vi "Main.vi"() -> ()   [LabVIEW 2017]
doc: "Use this template to build a user interface event handler design pattern. Use this pattern for dialog boxes and other user interfaces. You also can create and execute user-defined events that the VI can handle the same way as user interface events."
uses:
  <vilib>/Utility/NIReport.llb/HTML Report Image Alignment.ctl
  <vilib>/Utility/NIReport.llb/image depth.ctl
  <vilib>/addons/database/Connection.llb/DB Tools Open Connec (Path).vi
  <vilib>/addons/database/Auxilliary.llb/DB Tools Format Datetime String (Time Stamp).vi
  GLOBAL/auto.vi
  <vilib>/Utility/NIReport.llb/Append Report Text (str wrap).vi
  <vilib>/Utility/NIReport.llb/NI_report.lvclass
  <vilib>/addons/database/NI_Database_API.lvlib
  <vilib>/Utility/NIReport.llb/NI_ReportGenerationCore.lvlib
  <vilib>/Utility/NIReport.llb/Excel/NI_Excel.lvclass
panel:
  out "columns":string[](array[string])
  in  "MAX MIN VALUES":enum32{"ACTUAL", "SET"}(tab)
  out "TEMP":cluster{"MIN":dbl, "MAX":dbl, "ACTUAL":dbl}
  out "FLOW":cluster{"MIN":dbl, "MAX":dbl, "ACTUAL":dbl}
  out "BMP":cluster{"ACTUAL":dbl}
  out "Pressure":cluster{"MIN":dbl, "MAX":dbl, "ACTUAL":dbl}
  out "TEMP SET":cluster{"MIN":dbl, "MAX":dbl, "THRESHOLD":dbl}
  out "FLOW SET":cluster{"MIN":dbl, "MAX":dbl, "THRESHOLD":dbl}
  out "BMP SET":cluster{"MIN":dbl, "MAX":dbl, "THRESHOLD":dbl}
  out "Pressure SET":cluster{"MIN":dbl, "MAX":dbl, "THRESHOLD":dbl}
  out "Loading....":u8(slide) scale=0.0..100.0
  out "BMP":bool
  out "Temp":bool
  out "Flow":bool
  out "Pressure":bool
  in  "Generate Report":bool
  out "DESCRIPTION":string
  out "resulting string":path
  in  "import state 3":bool
  out "User Name":string
  out "Min Peak/Min":dbl
  out "Status bar":string
  in  "import state 2":bool
  out "SELECTED RECIPE":string
  out "BARCODE_FOUND":bool
  out "DB CONN":bool
  in  "Graph":bool
  out "table":string[][](table)
  out "GRAPH":cluster{timestamp[], ext[]}[](graph)
  out "TEST RESULT":bool
  in  "BARCODE":string
  out "SELECTED FILE PATH":path
  in  "Import File":bool
  in  "SELECT MEASURED FILE":i32(listbox)
  out "error out":errorcluster
  in  "File Name":string
  in  "Report Files Folder":path
  in  "Convert":bool
  in  "BROWSE FILE FOLDER":path
  in  "stop":bool
  # "Main"
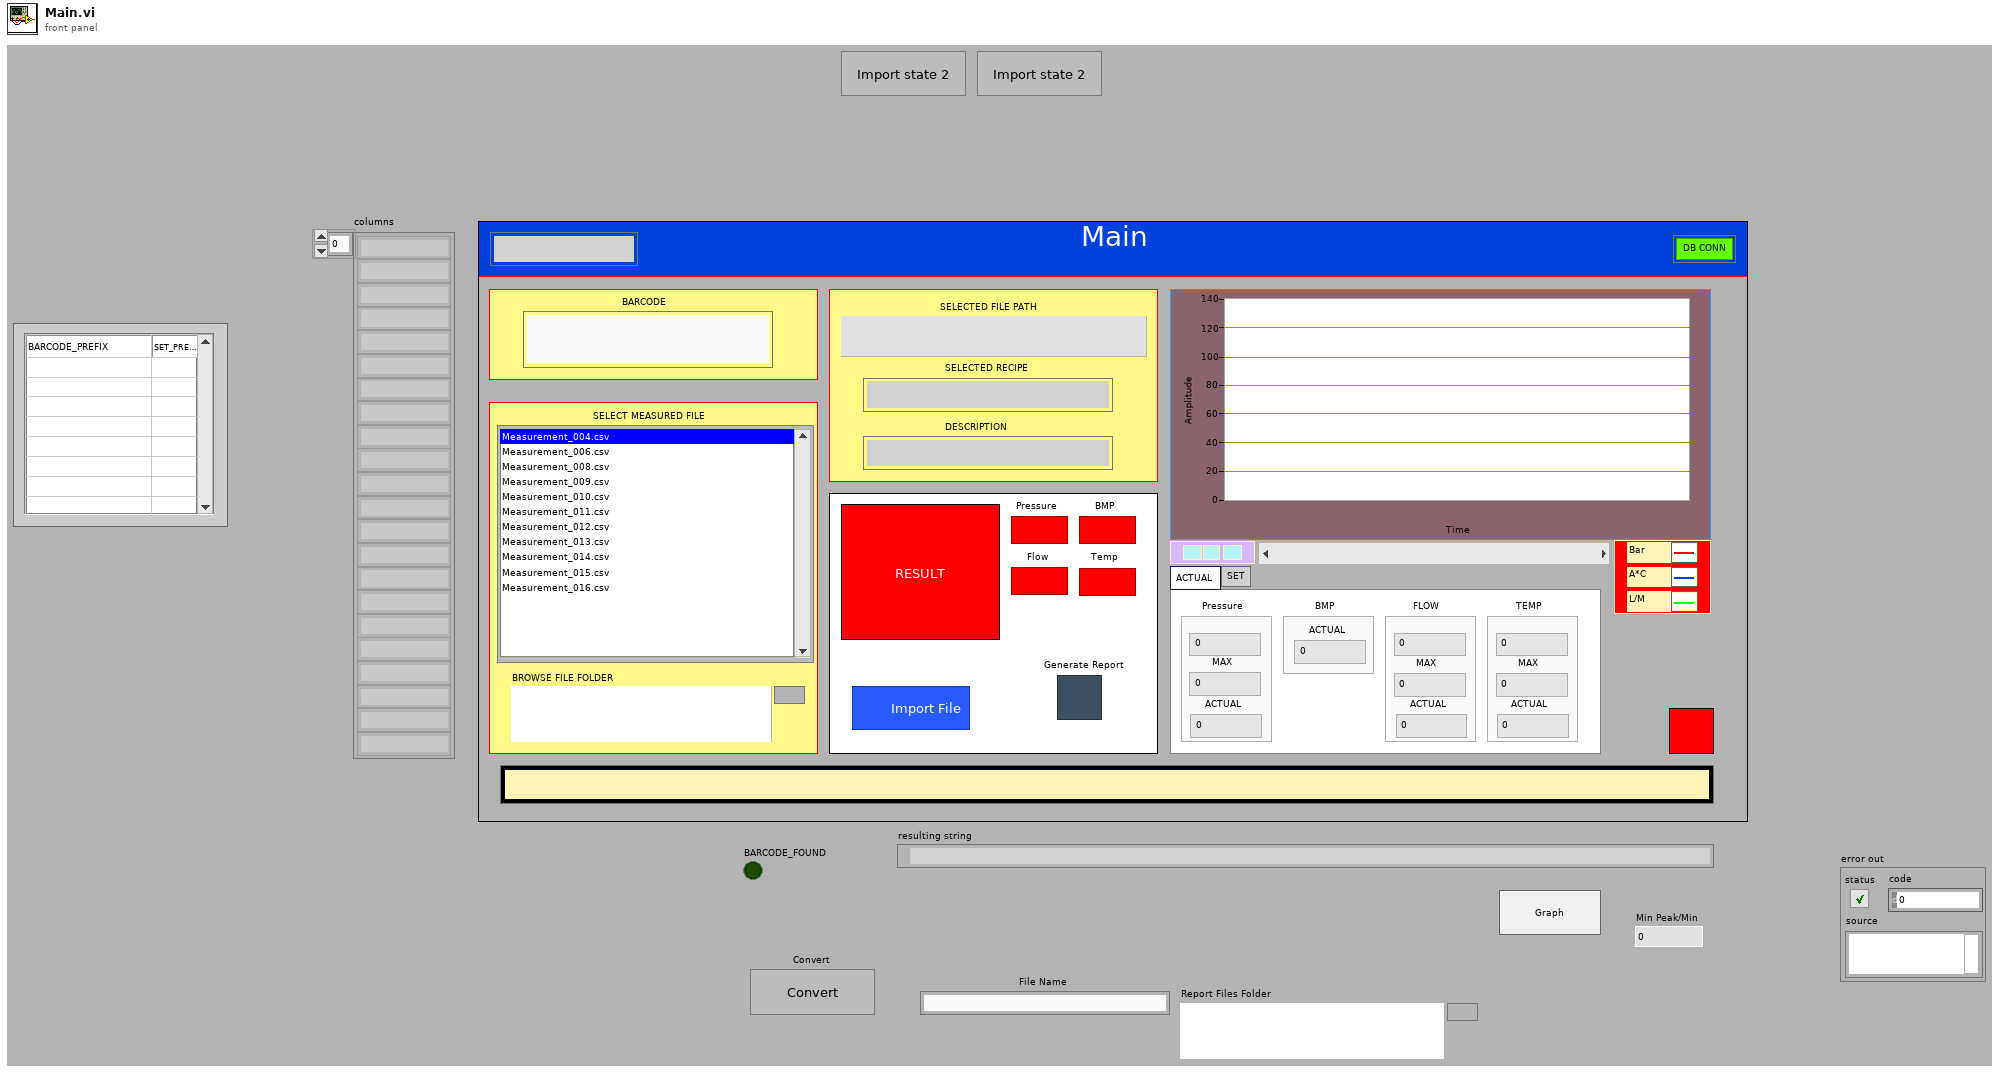
[diagram p1: front panel]
types:
  T1 = cluster{"Files":string[], "Browse File":path, "TIMEOUT":i32, "GRAPH":cluster{timestamp[], ext[]}[], "Pressure":cluster{"chl1 MIN":dbl, "chl1 MAX":dbl, "chl1 thrshold":dbl}, "Flow":cluster{"chl2 MIN":dbl, "chl2 MAX":dbl, "chl2 thrshold":dbl}, "Temp":cluster{"chl3 MIN":dbl, "chl3 MAX":dbl, "chl3 thrshold":dbl}, "Report File":path, "Data_to_report":cluster{"date/time string":string, "User Name":string, "BARCODE":string, "SELECTED RECIPE":string, "Rst":string, "Error Code":string, "RESULT ARRAY":string[]}, "BMP":cluster{"chl3 MIN":dbl, "chl3 MAX":dbl, "chl3 thrshold":dbl}}
  T2 = typedef "NI_Database_API.lvlib/Conn ObjectReference.ctl" = refnum<k1>
  T3 = enum32{"Invalid", "Standard", "Closed", "Hidden", "Minimized", "Maximized"}
  T4 = cluster{"position (Excel)":cluster{"row":i32, "column":i32}, "name (Excel)":string, "bookmark (Word)":string}[]
  T5 = cluster{"position (Excel)":cluster{"row":i32, "column":i32}, "name (Excel)":string, "bookmark (Word)":string}
  T6 = typedef "NI_ReportGenerationCore.lvlib/HTML Report Image Alignment.ctl" = enum16{"(default)", "LEFT", "RIGHT", "TOP", "TEXTTOP", "MIDDLE", "ABSMIDDLE", "BASELINE", "BOTTOM", "ABSBOTTOM"}
  T7 = enum16{"Standard Report", "HTML", "Word", "Excel"}
  T8 = enum16{"maximized", "minimized", "normal", "no change"}
  T9 = cluster{"Pressure":cluster{"chl1 MIN":dbl, "chl1 MAX":dbl, "chl1 thrshold":dbl}, "Flow":cluster{"chl2 MIN":dbl, "chl2 MAX":dbl, "chl2 thrshold":dbl}, "Temp":cluster{"chl3 MIN":dbl, "chl3 MAX":dbl, "chl3 thrshold":dbl}, "BMP":cluster{"chl3 MIN":dbl, "chl3 MAX":dbl, "chl3 thrshold":dbl}}
  T10 = cluster{"chl1 MIN":dbl, "chl1 MAX":dbl, "chl1 thrshold":dbl}
  T11 = cluster{"chl2 MIN":dbl, "chl2 MAX":dbl, "chl2 thrshold":dbl}
  T12 = cluster{"chl3 MIN":dbl, "chl3 MAX":dbl, "chl3 thrshold":dbl}
  T13 = cluster{"date/time string":string, "User Name":string, "BARCODE":string, "SELECTED RECIPE":string, "Rst":string, "Error Code 2":string}
  T14 = cluster{"date/time string":string, "User Name":string, "BARCODE":string, "SELECTED RECIPE":string, "Rst":string, "Error Code 2":string, "element":string, "element":string, "element":string, "element":string, "element":string, "element":string, "element":string, "element":string, "element":string, "element":string, "element":string}
  T15 = cluster{"date/time string":string, "User Name":string, "BARCODE":string, "SELECTED RECIPE":string, "Rst":string, "Error Code 2":string, "RESULT ARRAY":string[]}
  T16 = typedef "NI_ReportGenerationCore.lvlib/image depth.ctl" = u16
  T17 = enum32{"invalid app kind", "Development System", "Run Time System", "Student Edition", "Embedded LabVIEW", "Evaluation", "Custom"}
  T18 = cluster{"date/time string":string, "User Name":string, "BARCODE":string, "SELECTED RECIPE":string, "Rst":string, "Error Code":string, "RESULT ARRAY":string[]}
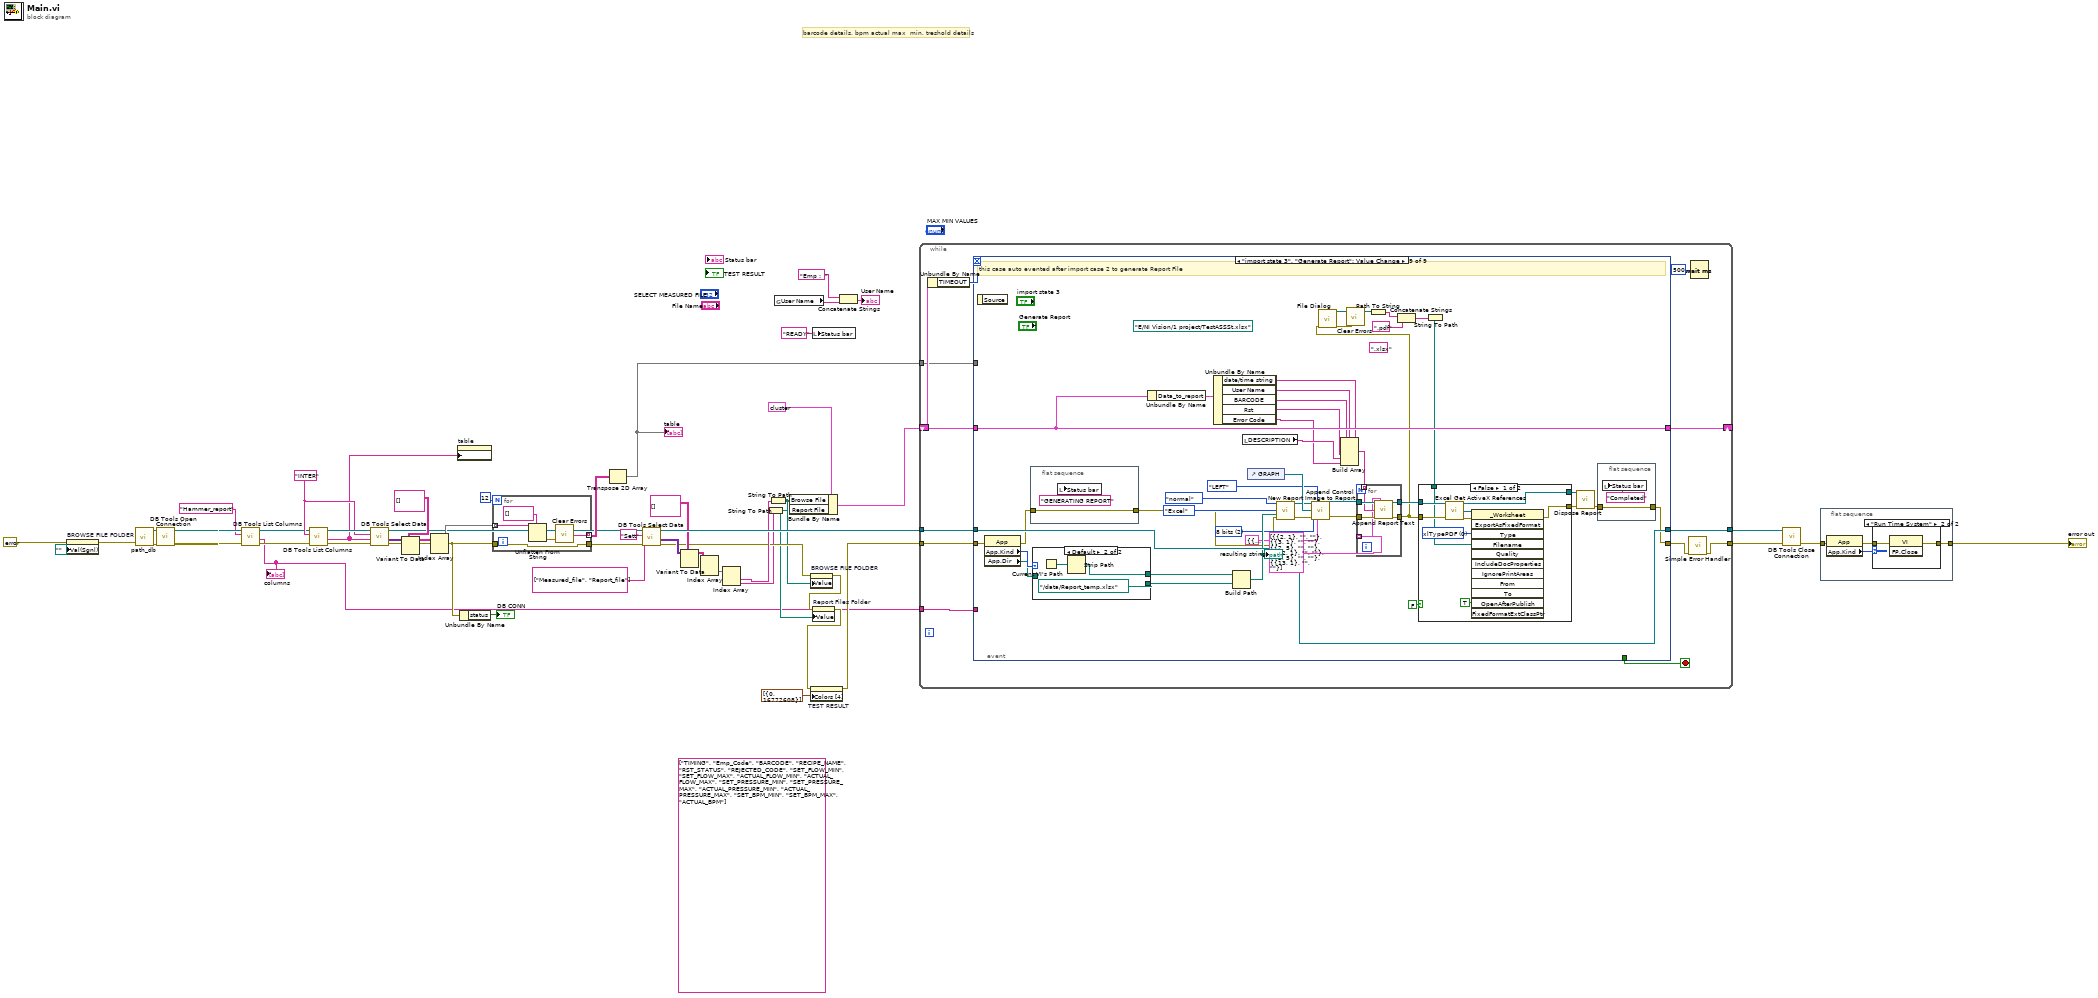
[diagram p0: block diagram]
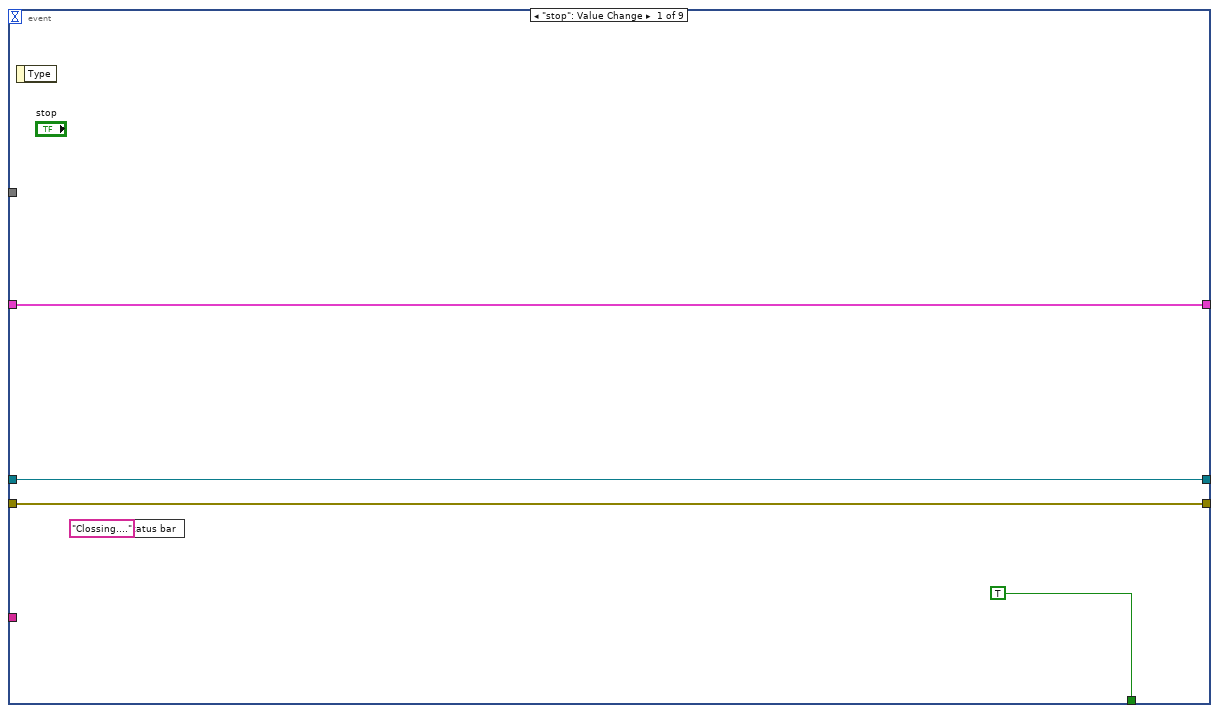
[diagram p3: hidden frame]
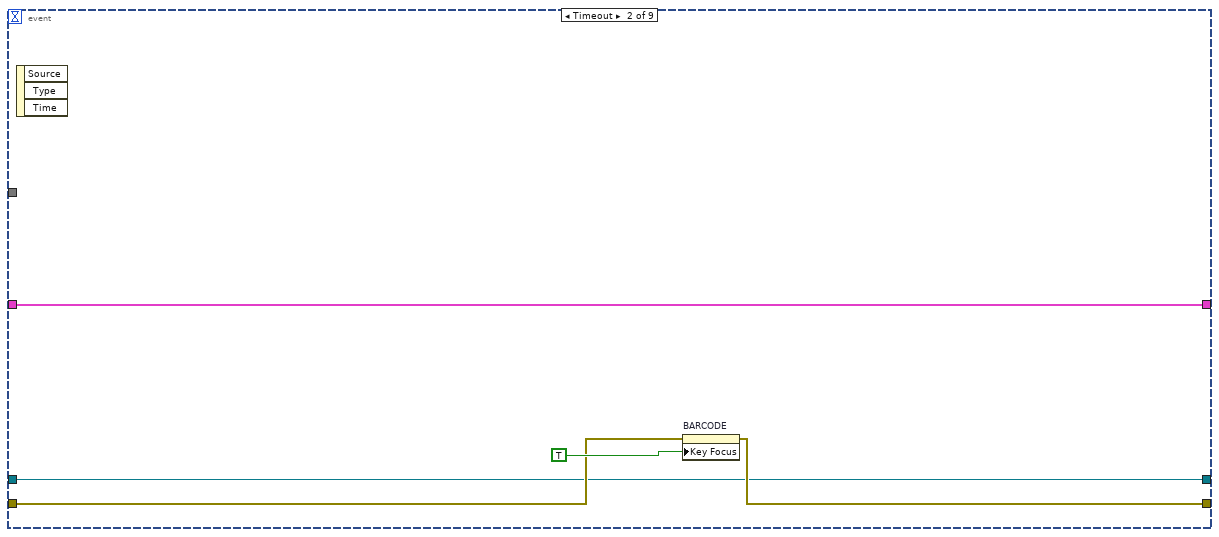
[diagram p4: hidden frame]
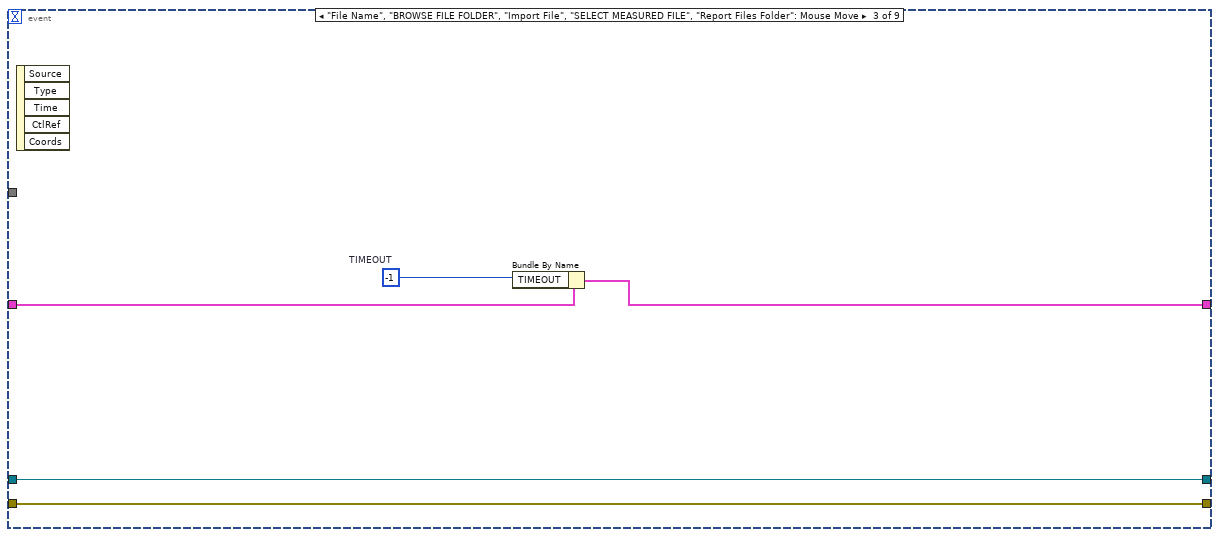
[diagram p5: hidden frame]
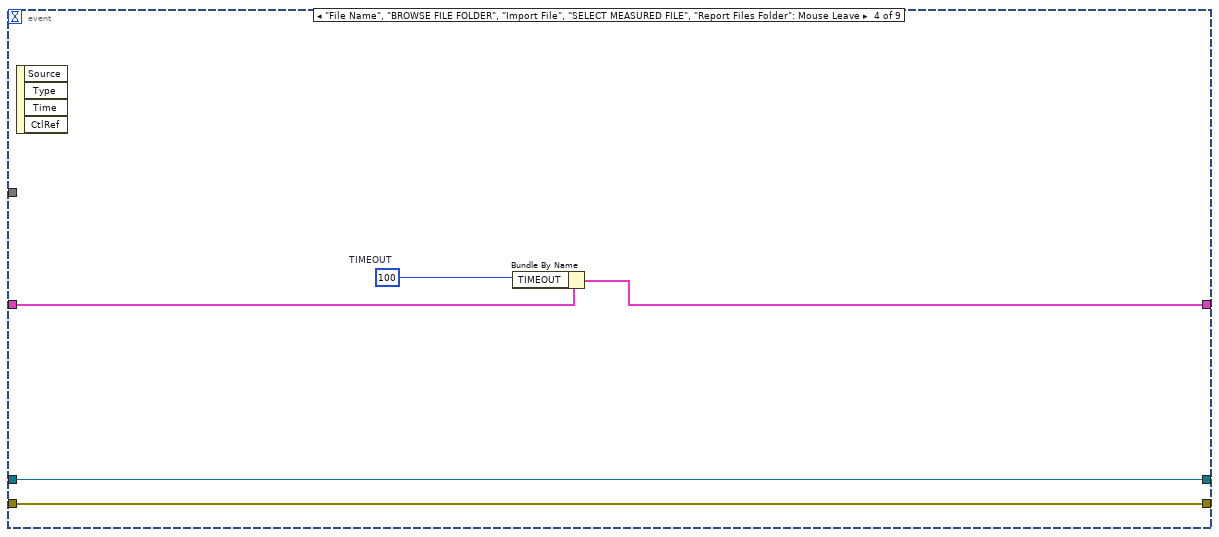
[diagram p6: hidden frame]
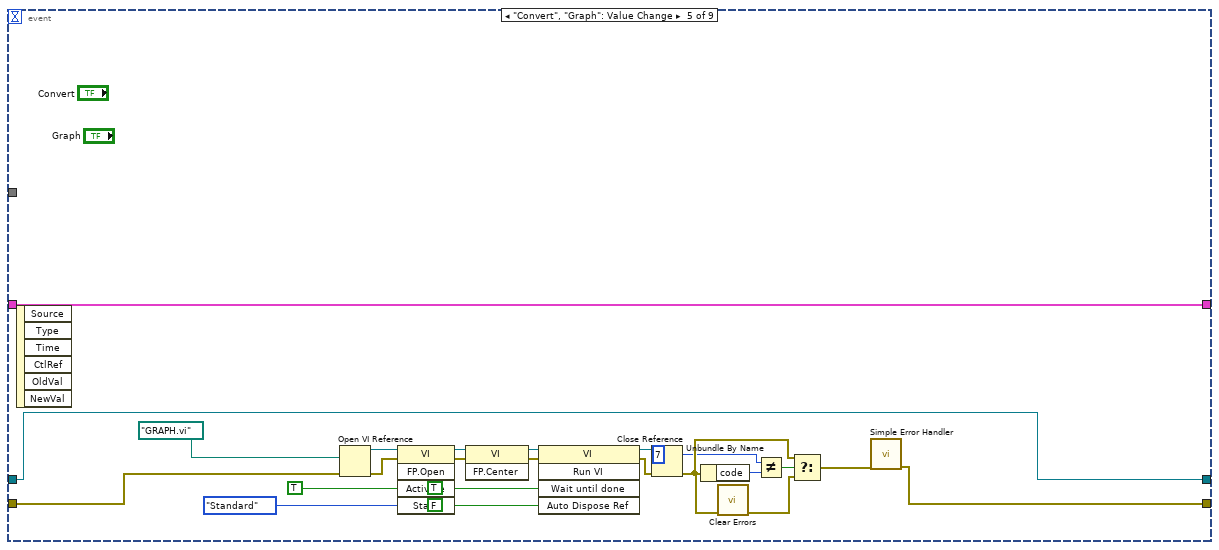
[diagram p7: hidden frame]
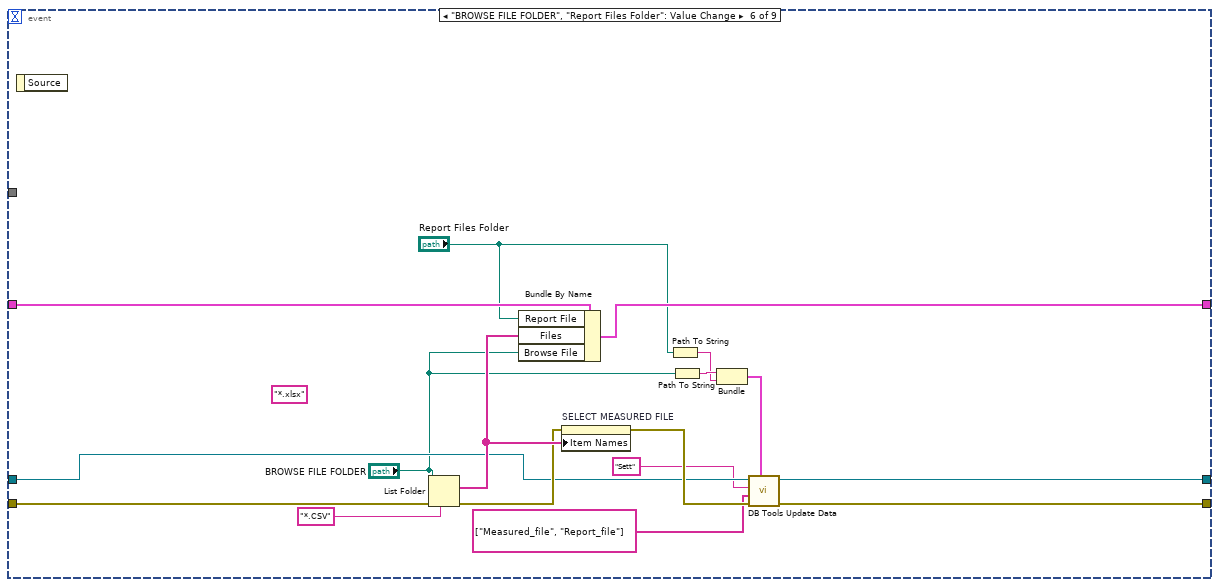
[diagram p8: hidden frame]
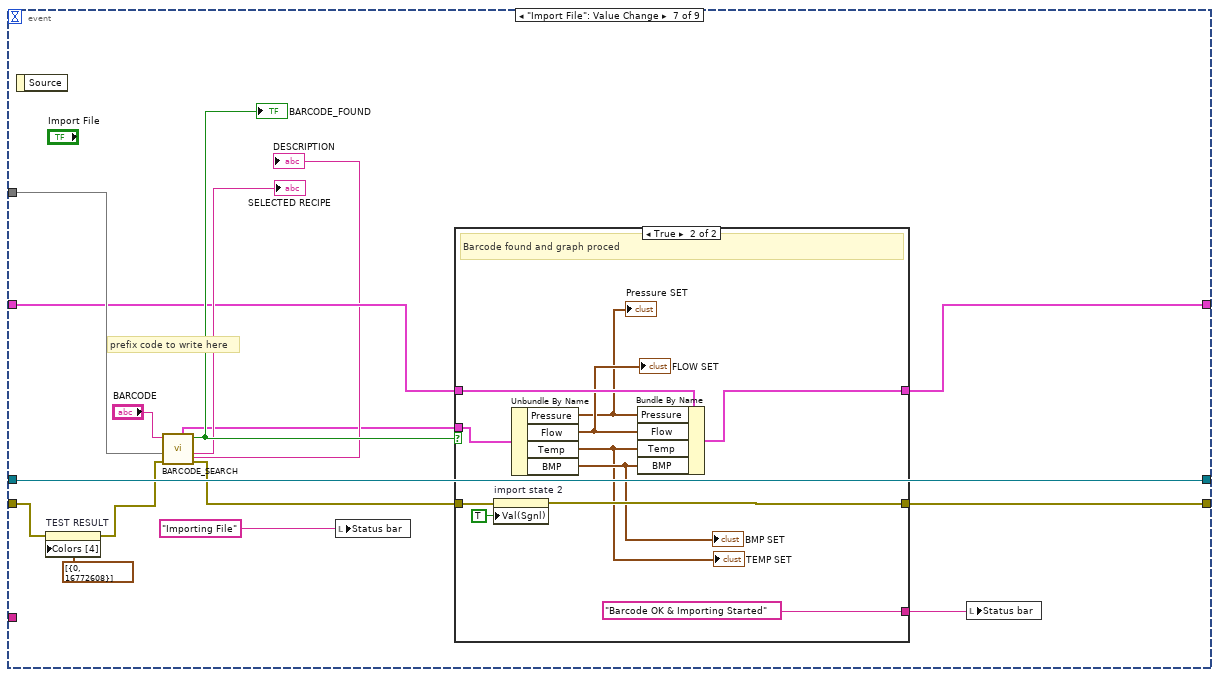
[diagram p9: hidden frame]
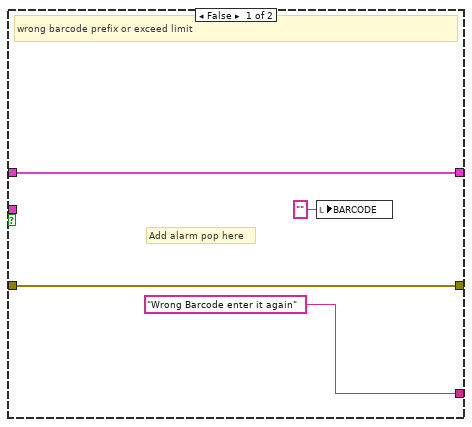
[diagram p10: hidden frame]
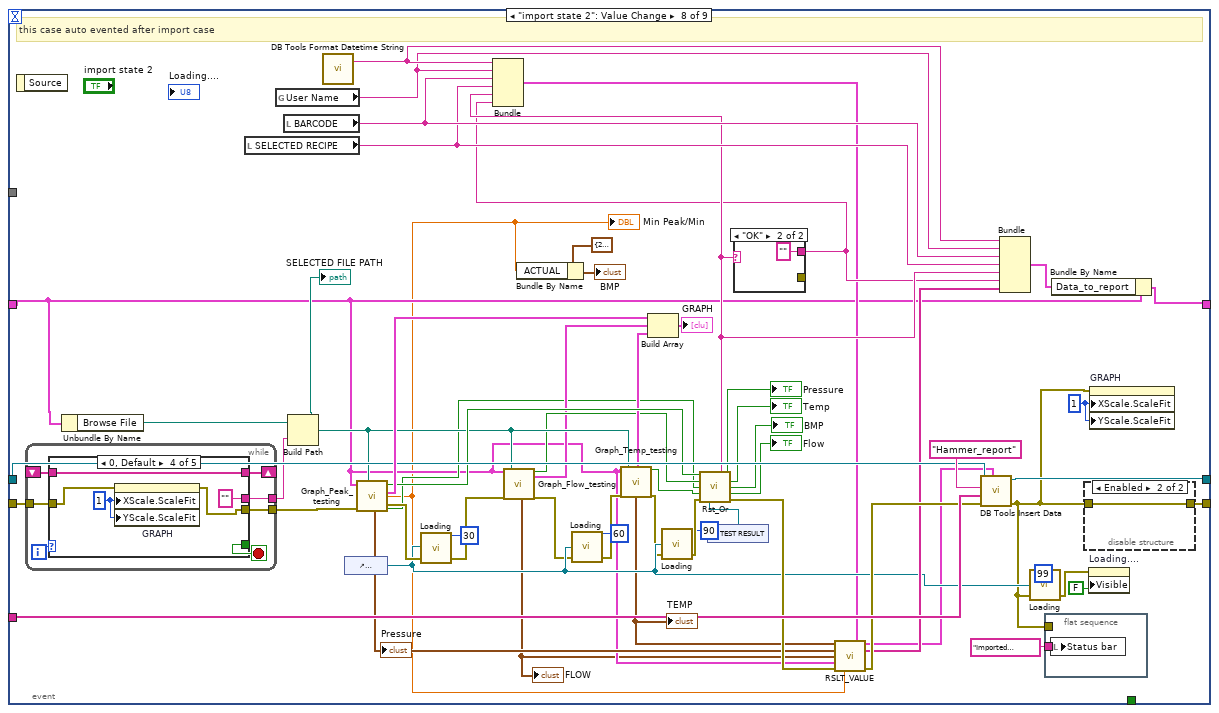
[diagram p11: hidden frame]
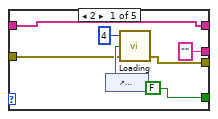
[diagram p12: hidden frame]
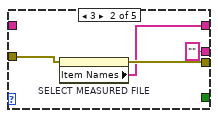
[diagram p13: hidden frame]
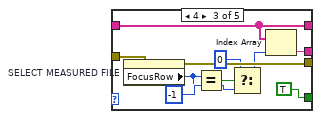
[diagram p14: hidden frame]
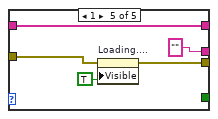
[diagram p15: hidden frame]
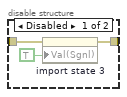
[diagram p16: hidden frame]
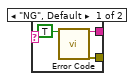
[diagram p17: hidden frame]
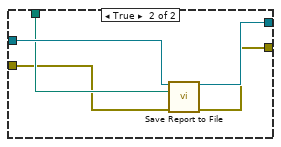
[diagram p18: hidden frame]
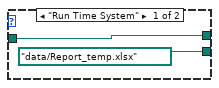
[diagram p19: hidden frame]
diagram:
  (unwired) string[] ["TIMING", "Emp_Code", "BARCODE", "RECIPE_NAME", "RST_STATUS", "REJECTED_CODE", "SET_FLOW_MIN", "SET_FLOW_MAX", "ACTUAL_FLOW_MIN", "ACTUAL_FLOW_MAX", "SET_PRESSURE_MIN", "SET_PRESSURE_MAX", "ACTUAL_PRESSURE_MIN", "ACTUAL_PRESSURE_MAX", "SET_BPM_MIN", "SET_BPM_MAX", "ACTUAL_BPM"] ("columns")
  w11 = "INTER" ("table")
  # "barcode details, bpm actual max  min, treshold details"
  n1 = property on="BROWSE FILE FOLDER" class="Path"(error in=errorcluster {"status"=FALSE, "code"=0, "source"=""} ("error out 2"), "Val(Sgnl)"=path "" ("BROWSE FILE FOLDER")) -> (error out=w25:errorcluster)  [unwired: 1 in, 1 out]
  n2 = call "path_db.vi"("error in"=w25) -> ("error out"=w49:errorcluster, "resulting string"=w48:path)  [unwired: 9 in]
  n3 = call-poly <vilib>:"DB Tools Open Connection.vi"("error in (no error)"=w49, "connection information"=w48) -> ("error out"=w9:errorcluster, "connection reference"=w7:T2)  [unwired: 6 in]
  n4 = call <vilib>:"DB Tools List Columns.vi"("error in (no error)"=w9, "table"="Hammer_report", "connection reference"=w7) -> ("error out"=w8:errorcluster, "columns"=w4:string[], "connection reference out"=w6:T2)  [unwired: 1 in, 1 out]
  "columns" <- w4
  n5 = call <vilib>:"DB Tools List Columns.vi"("error in (no error)"=w8, "table"=w11, "connection reference"=w6) -> ("error out"=w13:errorcluster, "columns"=w1:string[], "connection reference out"=w12:T2)  [unwired: 1 in, 1 out]
  n6 = call <vilib>:"DB Tools Select Data.vi"("error in (no error)"=w13, "columns"=w1, "table"=w11, "connection reference"=w12) -> ("error out"=w43:errorcluster, "data"=w51:variant[][], "connection reference out"=w38:T2)  [unwired: 2 in]
  n7 = Variant To Data(type=string[][] [], Variant=w51) -> (data=w50:string[][])  [unwired: 1 in, 1 out]
  n8 = Index Array(array=w50) -> (element=w46:string[])  [unwired: 2 in]
  n9 = property on="table" class="Tbl (strict)"("Column Headers[]"=w1) -> ()  [unwired: 2 in, 2 out]
  n10 = Unbundle By Name(w43) -> ("status"=→"DB CONN":bool)
  n11 = for {
    N: 12 -> [_]
    tunnel: w46 -> [w56] mode=indexing
    tunnel: [w54] -> w45 mode=indexing
    tunnel: w43 -> [w53]
    tunnel: [w53] -> w39
    n12 = Unflatten From String(type=string[] [], binary string=w56) -> (value=w54:string[], error out=w57:errorcluster)  [unwired: 3 in, 1 out]
    n13 = call <vilib>:"Clear Errors.vi"("error in (no error)"=w57) -> ()  [unwired: 5 in, 2 out]
  }
  n14 = Transpose 2D Array(2D array=w45) -> (transposed array=w23:string[][])
  "table" <- w23
  n15 = call <vilib>:"DB Tools Select Data.vi"("error in (no error)"=w39, "columns"=string[] ["Measured_file", "Report_file"], "table"="Sett", "connection reference"=w38) -> ("error out"=w28:errorcluster, "data"=w36:variant[][], "connection reference out"=w37:T2)  [unwired: 2 in]
  n16 = Variant To Data(type=string[][] [], Variant=w36) -> (data=w34:string[][])  [unwired: 1 in, 1 out]
  n17 = Index Array(array=w34) -> (element=w30:string[])  [unwired: 2 in]
  n18 = Index Array(array=w30) -> (element #1=w29:string, element #2=w22:string)  [unwired: 2 in]
  n19 = String To Path(string=w22) -> (path=w21:path)
  n20 = String To Path(string=w29) -> (path=w27:path)
  n21 = global read "auto.vi" "User Name"() -> (w3:string)
  n22 = Bundle By Name(cluster=T1 {"Files"=[], "Browse File"=path "", "TIMEOUT"=100, "GRAPH"=[{array[68443 elements], array[68443 elements]}, {array[68363 elements], array[68363 elements]}, {array[40500 elements], array[40500 elements]}], "Pressure"={"chl1 MIN"=110.0, "chl1 MAX"=130.0, "chl1 thrshold"=120.0}, "Flow"={"chl2 MIN"=33.0, "chl2 MAX"=35.0, "chl2 thrshold"=25.0}, "Temp"={"chl3 MIN"=20.0, "chl3 MAX"=30.0, "chl3 thrshold"=34.0}, "Report File"=path "", "Data_to_report"={"date/time string"="", "User Name"="", "BARCODE"="", "SELECTED RECIPE"="", "Rst"="", "Error Code"="", "RESULT ARRAY"=[]}, "BMP"={"chl3 MIN"=1000.0, "chl3 MAX"=2000.0, "chl3 thrshold"=0.0}}, "Browse File"=w27, "Report File"=w21) -> (w31:T1)
  n23 = property on="BROWSE FILE FOLDER" class="Path"(error in=w28, "Value"=w27) -> (error out=w20:errorcluster)  [unwired: 1 in, 1 out]
  n24 = local write "Status bar"("READY" ("Status bar")) -> ()
  n25 = property on="Report Files Folder" class="Path"(error in=w20, "Value"=w21) -> (error out=w19:errorcluster)  [unwired: 1 in, 1 out]
  n26 = property on="TEST RESULT" class="Bool"(error in=w19, "Colors [4]"=cluster{u32, u32}[] [{0, 16772608}]) -> (error out=w15:errorcluster)  [unwired: 1 in, 1 out]
  n27 = Concatenate Strings("Emp :  " ("string"), w3) -> (→"User Name":string)
  n28 = while {
    tunnel: w15 -> [w67]
    tunnel: [w59] -> w42
    shift-right: [w66] -> _
    shift-left: w31 -> [w64]
    tunnel: w37 -> [w62]
    tunnel: [w63] -> w41
    tunnel: w23 -> [w61]
    tunnel: w4 -> [w58]
    stop <- w69 stop-if-true
    n29 = Unbundle By Name(w64) -> ("TIMEOUT"=w65:i32)
    n30 = event shown="[8] \"import state 3\", \"Generate Report\": Value Change" {
      selector: _ -> [_ _ _ _ _ _ _ _ _]
      dyn-events: _ -> [_ _ _ _ _ _ _ _ _]
      timeout: w65 -> [_ _ _ _ _ _ _ _ _]
      tunnel: [TRUE _ _ _ _ _ _ _ _] -> w69
      tunnel: w67 -> [w73 w77 w84 w89 w92 w129 w135 w196 w303]
      tunnel: [w73 w76 w84 w89 w91 w122 w142 w213 w285] -> w60
      tunnel: w64 -> [w74 w79 w83 w88 w112 w128 w138 w167 w291]
      tunnel: [w74 w79 w82 w87 w112 w127 w137 w212 w291] -> w66
      tunnel: [w71 w75 w80 w85 w90 w120 w145 w214 w308] -> w63
      tunnel: w62 -> [w71 w75 w80 w85 w90 w121 w145 w215 w308]
      tunnel: w61 -> [_ _ _ _ _ _ w139 _ _]
      tunnel: w58 -> [_ _ _ _ _ _ _ w210 _]
      event "stop": Value Change {
        n31 = event-data() -> ()  [unwired: 1 in, 1 out]
        n32 = local write "Status bar"("Clossing...." ("Status bar")) -> ()
      }
      event Timeout {
        n33 = event-data() -> ()  [unwired: 1 in, 3 out]
        n34 = property on="BARCODE" class="Str"(error in=w77, "Key Focus"=TRUE) -> (error out=w76:errorcluster)  [unwired: 1 in, 1 out]
      }
      event "File Name", "BROWSE FILE FOLDER", "Import File", "SELECT MEASURED FILE", "Report Files Folder": Mouse Move {
        w81 = -1  # TIMEOUT
        n35 = event-data() -> ()  [unwired: 1 in, 5 out]
        n36 = Bundle By Name(cluster=w83, "TIMEOUT"=w81) -> (w82:T1)
      }
      event "File Name", "BROWSE FILE FOLDER", "Import File", "SELECT MEASURED FILE", "Report Files Folder": Mouse Leave {
        w86 = 100  # TIMEOUT
        n37 = event-data() -> ()  [unwired: 1 in, 4 out]
        n38 = Bundle By Name(cluster=w88, "TIMEOUT"=w86) -> (w87:T1)
      }
      event "Convert", "Graph": Value Change {
        n39 = event-data() -> ()  [unwired: 1 in, 6 out]
        n40 = Open VI Reference(vi path=path "GRAPH.vi", error in (no error)=w92) -> (vi reference=w99:refnum<vi>, error out=w111:errorcluster)  [unwired: 4 in]
        n41 = invoke class="VI" method="FP.Open"(reference=w99, error in=w111, "Activate"=TRUE ("Activate?"), "State"=T3."Standard") -> (reference out=w110:refnum<vi>, error out=w105:errorcluster)  [unwired: 1 in, 3 out]
        n42 = invoke class="VI" method="FP.Center"(reference=w110, error in=w105) -> (reference out=w106:refnum<vi>, error out=w107:errorcluster)  [unwired: 1 in, 1 out]
        n43 = invoke class="VI" method="Run VI"(reference=w106, error in=w107, "Wait until done"=TRUE ("Wait Until Done"), "Auto Dispose Ref"=FALSE ("Auto Dispose Reference")) -> (reference out=w108:refnum<vi>, error out=w109:errorcluster)  [unwired: 1 in, 3 out]
        n44 = Close Reference(reference=w108, error in (no error)=w109) -> (error out=w100:errorcluster)
        n45 = Unbundle By Name(w100) -> ("code"=w104:i32)
        n46 = call <vilib>:"Clear Errors.vi"("error in (no error)"=w100) -> ("error out"=w102:errorcluster)  [unwired: 5 in, 1 out]
        n47 = Not Equal?(x=7, y=w104) -> (x != y?=w103:bool)
        n48 = Select(t=w100, s=w103, f=w102) -> (s? t:f=w101:errorcluster)
        n49 = call <vilib>:"Simple Error Handler.vi"("error in (no error)"=w101) -> ("error out"=w91:errorcluster)  [unwired: 4 in, 4 out]
      }
      event "BROWSE FILE FOLDER", "Report Files Folder": Value Change {
        (unwired) "*.xlsx" ("pattern")
        n50 = event-data() -> ()  [unwired: 1 in, 1 out]
        n51 = List Folder(path="BROWSE FILE FOLDER", pattern="*.CSV", error in=w129) -> (filenames=w125:string[], error out=w124:errorcluster)  [unwired: 1 in, 2 out]
        n52 = Bundle By Name(cluster=w128, "Report File"="Report Files Folder", "Files"=w125, "Browse File"="BROWSE FILE FOLDER") -> (w127:T1)
        n53 = property on="SELECT MEASURED FILE" class="LstBox (strict)"(error in=w124, "Item Names"=w125) -> (error out=w123:errorcluster)  [unwired: 1 in, 1 out]
        n54 = Path To String(path="Report Files Folder") -> (string=w114:string)
        n55 = Path To String(path="BROWSE FILE FOLDER") -> (string=w116:string)
        n56 = Bundle(w116, w114) -> (w119:cluster{string, string})  [unwired: 1 in]
        n57 = call <vilib>:"DB Tools Update Data.vi"("data"=w119, "error in (no error)"=w123, "columns"=string[] ["Measured_file", "Report_file"], "table"="Sett", "connection reference"=w121) -> ("error out"=w122:errorcluster, "connection reference out"=w120:T2)  [unwired: 5 in]
      }
      event "Import File": Value Change {
        # "prefix code to write here"
        n58 = event-data() -> ()  [unwired: 1 in, 1 out]
        n59 = property on="TEST RESULT" class="Bool"(error in=w135, "Colors [4]"=cluster{u32, u32}[] [{0, 16772608}]) -> (error out=w134:errorcluster)  [unwired: 1 in, 1 out]
        n60 = call "BARCODE_SEARCH.vi"("error in"=w134, "BARCODE_TABLE"=w139, "BARCODE_TO_SEARCH"="BARCODE") -> ("error out"=w143:errorcluster, "ARTICLE name"=→"SELECTED RECIPE":string, "BARCODE_FOUND"=w141:bool, "description NAME"=→"DESCRIPTION":string, "CHL"=w130:T9)  [unwired: 3 in, 1 out]
        "BARCODE_FOUND" <- w141
        n61 = local write "Status bar"("Importing File" ("Status bar")) -> ()
        n62 = case shown="True" w141 {
          tunnel: [w149 w158] -> w142
          tunnel: w143 -> [w149 w159]
          tunnel: [w148 w156] -> w137
          tunnel: w138 -> [w148 w157]
          tunnel: ["Wrong Barcode enter it again" ("Status bar") "Barcode OK & Importing Started" ("Status bar")] -> w132
          tunnel: w130 -> [_ w154]
          frame False {
            # "Add alarm pop here"
            # "wrong barcode prefix or exceed limit"
            n63 = local write "BARCODE"("" ("BARCODE")) -> ()
          }
          frame True {
            # "Barcode found and graph proced"
            n64 = property on="import state 2" class="Bool (strict)"(error in=w159, "Val(Sgnl)"=TRUE) -> (error out=w158:errorcluster)  [unwired: 1 in, 1 out]
            n65 = Unbundle By Name(w154) -> ("Pressure"=w150:T10, "Flow"=w153:T11, "Temp"=w151:T12, "BMP"=w152:T12)
            "Pressure SET" <- w150
            "BMP SET" <- w152
            "FLOW SET" <- w153
            "TEMP SET" <- w151
            n66 = Bundle By Name(cluster=w157, "Pressure"=w150, "Flow"=w153, "Temp"=w151, "BMP"=w152) -> (w156:T1)
          }
        }
        n67 = local write "Status bar"(w132) -> ()
      }
      event "import state 2": Value Change {
        w163 = u8 1 ("X Scale.Scale Fit")
        # "this case auto evented after import case"
        n68 = event-data() -> ()  [unwired: 1 in, 1 out]
        n69 = while {
          tunnel: [w226] -> w195
          tunnel: w196 -> [w225]
          shift-right: [w222] -> _
          shift-left: _ -> [w221]
          tunnel: [w220] -> w194
          i -> [w224]
          stop <- w223 stop-if-true
          n70 = case shown="0, Default" w224 {
            tunnel: [w231 w237 w246 w249 w256] -> w226
            tunnel: w225 -> [w230 w236 w247 w248 w255]
            tunnel: [FALSE _ TRUE _ _] -> w223
            tunnel: [w228 w235 w240 w251 w254] -> w222
            tunnel: w221 -> [w228 _ w240 w251 w254]
            tunnel: ["" "" w239 "" ""] -> w220
            frame 2 {
              n71 = control-ref of="Loading...."() -> (w233:refnum<vi>)
              n72 = call "Loading.vi"("error in"=w230, "reference"=w233, "Value"=u8 4) -> ("error out"=w231:errorcluster)  [unwired: 2 in]
            }
            frame 3 {
              n73 = property on="SELECT MEASURED FILE" class="LstBox (strict)"(error in=w236) -> (error out=w237:errorcluster, "Item Names"=w235:string[])  [unwired: 1 in, 1 out]
            }
            frame 4 {
              n74 = property on="SELECT MEASURED FILE" class="LstBox (strict)"(error in=w247) -> (error out=w246:errorcluster, "FocusRow"=w242:i32)  [unwired: 1 in, 1 out]
              n75 = Equal?(x=w242, y=-1) -> (x = y?=w245:bool)
              n76 = Select(t=0 ("y"), s=w245, f=w242) -> (s? t:f=w241:i32)
              n77 = Index Array(array=w240, index=w241) -> (element=w239:string)
            }
            frame 0, Default {
              w252 = u8 1 ("X Scale.Scale Fit")
              n78 = property on="GRAPH" class="XYGraph (strict)"(error in=w248, "XScale.ScaleFit"=w252, "YScale.ScaleFit"=w252) -> (error out=w249:errorcluster)  [unwired: 1 in, 1 out]
            }
            frame 1 {
              n79 = property on="Loading...." class="Slide (strict)"(error in=w255, "Visible"=TRUE) -> (error out=w256:errorcluster)  [unwired: 1 in, 1 out]
            }
          }
        }
        n80 = Unbundle By Name(w167) -> ("Browse File"=w219:path)
        n81 = local read "SELECTED RECIPE"() -> (w173:string)
        n82 = global read "auto.vi" "User Name"() -> (w175:string)
        n83 = local read "BARCODE"() -> (w174:string)
        n84 = Build Path(base path=w219, name or relative path=w194) -> (appended path=w189:path)
        "SELECTED FILE PATH" <- w189
        n85 = call-poly <vilib>:"DB Tools Format Datetime String.vi"() -> ("date/time string"=w176:string)  [unwired: 1 in]
        n86 = control-ref of="Loading...."() -> (w199:refnum<vi>)
        n87 = call "Graph_Peak_testing.vi"("CSV file path"=w189, "error in"=w195, "Cluster"=w167) -> ("MIN_MAX_BPM"=w178:bool, "Filter Graph"=w217:cluster{timestamp[], ext[]}, "MIN_MAX_PRESSURE"=w197:bool, "ACTUAL BPM"=w161:dbl, "error out"=w203:errorcluster, "MAX_MIN_PRESSURE"=w181:cluster{"MIN":dbl, "MAX":dbl, "ACTUAL":dbl})  [unwired: 1 in, 1 out]
        "Min Peak/Min" <- w161
        "Pressure" <- w181
        n88 = call "Loading.vi"("error in"=w203, "reference"=w199, "Value"=u8 30) -> ("error out"=w187:errorcluster)  [unwired: 2 in]
        n89 = call "Graph_Flow_testing.vi"("Cluster"=w167, "error in"=w187, "CSV file path"=w189) -> ("MIN_MAX_FLOW"=w188:bool, "Filter Graph Flow"=w185:cluster{timestamp[], ext[]}, "MAX-MIN_Flow"=w166:cluster{"MIN":dbl, "MAX":dbl, "ACTUAL":dbl}, "error out"=w186:errorcluster)  [unwired: 13 in]
        "FLOW" <- w166
        n90 = Bundle By Name(cluster=cluster{"ACTUAL":dbl} {"ACTUAL"=21.503} ("BMP 2"), "ACTUAL"=w161) -> (→"BMP":cluster{"ACTUAL":dbl})
        n91 = call "Loading.vi"("error in"=w186, "reference"=w199, "Value"=u8 60) -> ("error out"=w193:errorcluster)  [unwired: 2 in]
        n92 = call "Graph_Temp_testing.vi"("Cluster"=w167, "error in"=w193, "CSV file path"=w189) -> (14:"MAX-MIN_Temp"=w191:bool, "Filter Graph"=w192:cluster{timestamp[], ext[]}, 16:"MAX-MIN_Temp"=w165:cluster{"MIN":dbl, "MAX":dbl, "ACTUAL":dbl}, "error out"=w190:errorcluster)  [unwired: 13 in]
        "TEMP" <- w165
        n93 = Build Array(w217, w185, w192) -> (→"GRAPH":cluster{timestamp[], ext[]}[])
        n94 = call "Loading.vi"("error in"=w190, "reference"=w199, "Value"=u8 90) -> ("error out"=w202:errorcluster)  [unwired: 2 in]
        n95 = control-ref of="TEST RESULT"() -> (w168:refnum<vi>)
        n96 = call "Rst_Or.vi"("BAR rst"=w197, "L/Min rst"=w188, "BPM rst"=w178, "A*C rst"=w191, "error In"=w202, "RST_COLOR"=w168) -> ("Rst"=w172:string, "BAR"=→"Pressure":bool, "L/Min"=→"Temp":bool, "BPM"=→"BMP":bool, "A*C"=→"Flow":bool, "error out"=w209:errorcluster)  [unwired: 4 in]
        n97 = case shown="\"OK\"" w172 {
          tunnel: [w265 ""] -> w171
          tunnel: [w264 _] -> _
          frame "NG", Default {
            n98 = call "Error Code.vi"("Enable"=TRUE) -> ("Error Code 2"=w265:string, "error out"=w264:errorcluster)  [unwired: 16 in, 1 out]
          }
          frame "OK" {
          }
        }
        n99 = Bundle("date/time string"=w176, "User Name"=w175, "BARCODE"=w174, "SELECTED RECIPE"=w173, "Rst"=w172, "Error Code 2"=w171) -> (w170:T13)  [unwired: 1 in]
        n100 = call "RSLT_VALUE.vi"("MAX-MIN Temp"=w165, "INPUT cluster"=w170, "MAX-MIN PRESSURE"=w181, "MAX-MIN FLOW"=w166, "CLUSTER"=w167, "error in"=w209, "ACTUAL BPM"=w161) -> ("CLUSTER TO SQL"=w169:T14, "RESULT ARRAY"=w207:string[], "error OUT"=w208:errorcluster)  [unwired: 6 in]
        n101 = call <vilib>:"DB Tools Insert Data.vi"("data"=w169, "error in (no error)"=w208, "columns"=w210, "table"="Hammer_report", "connection reference"=w215) -> ("error out"=w162:errorcluster, "connection reference out"=w214:T2)  [unwired: 5 in]
        n102 = Bundle("date/time string"=w176, "User Name"=w175, "BARCODE"=w174, "SELECTED RECIPE"=w173, "Rst"=w172, "Error Code 2"=w171, "RESULT ARRAY"=w207) -> (w206:T15)  [unwired: 1 in]
        n103 = call "Loading.vi"("error in"=w162, "reference"=w199, "Value"=u8 99) -> ("error out"=w164:errorcluster)  [unwired: 2 in]
        n104 = flat-sequence {
          tunnel: "Imported Completed & Click on Generate Report button for Report" ("Status bar") -> [w258]
          tunnel: w162 -> [_]
          frame #0 {
            n105 = local write "Status bar"(w258) -> ()
          }
        }
        n106 = Bundle By Name(cluster=w167, "Data_to_report"=w206) -> (w212:T1)
        n107 = disable-structure shown="Enabled" {
          disable-tunnel: w162 -> [w261 w262]
          disable-tunnel: [w260 w262] -> w213
          frame Disabled {
            n108 = property on="import state 3" class="Bool (strict)"(error in=w261, "Val(Sgnl)"=TRUE) -> (error out=w260:errorcluster)  [unwired: 1 in, 1 out]
          }
          frame Enabled {
          }
        }
        n109 = property on="Loading...." class="Slide (strict)"(error in=w164, "Visible"=FALSE) -> ()  [unwired: 1 in, 2 out]
        n110 = property on="GRAPH" class="XYGraph (strict)"(error in=w162, "XScale.ScaleFit"=w163, "YScale.ScaleFit"=w163) -> ()  [unwired: 1 in, 2 out]
      }
      event "import state 3", "Generate Report": Value Change {
        (unwired) ".xlsx" ("string")
        (unwired) path "E:/NI Vision/1 project/TestASSSt.xlsx" ("report file path")
        w292 = T16 2 items=["B&W", "4 bits", "8 bits", "24 bits"] ("image depth")
        # "this case auto evented after import case 2 to generate Report File"
        n111 = event-data() -> ()  [unwired: 1 in, 1 out]
        n112 = property class="App"(error in=w303) -> (error out=w287:errorcluster, "App.Kind"=w307:T17, "App.Dir"=w306:path)  [unwired: 1 in, 1 out]
        n113 = flat-sequence {
          tunnel: w287 -> [w331]
          tunnel: [w331] -> w286
          frame #0 {
            n114 = local write "Status bar"("GENERATING REPORT" ("Status bar")) -> ()
          }
        }
        n115 = case shown="Default" w307 {
          tunnel: w306 -> [w334 _]
          tunnel: [path "data/Report_temp.xlsx" ("path") path "../data/Report_temp.xlsx" ("path")] -> w305
          tunnel: [w334 w335] -> w304
          frame "Run Time System" {
          }
          frame Default {
            n116 = Current VI's Path() -> (path=w336:path)
            n117 = Strip Path(path=w336) -> (stripped path=w335:path)  [unwired: 1 out]
          }
        }
        n118 = Unbundle By Name(w291) -> ("Data_to_report"=w270:T18)
        n119 = Unbundle By Name(w270) -> ("date/time string"=w271:string, "User Name"=w272:string, "BARCODE"=w273:string, "Rst"=w274:string, "Error Code"=w268:string)
        n120 = Build Path(base path=w304, name or relative path=w305) -> (appended path=w297:path)
        "resulting string" <- w297
        n121 = local read "DESCRIPTION"() -> (w269:string)
        n122 = control-ref of="GRAPH"() -> (w300:refnum<vi>)
        n123 = call <vilib>:"New Report.vi"("window state (normal)"=T8."normal", "report type"=T7."Excel", "template (empty)"=w297, "error in (no error)"=w286) -> ("report out"=w299:refnum<class "NI_report.lvclass">, "error out"=w298:errorcluster)  [unwired: 10 in]
        n124 = call-dynamic "Append Control Image to Report.vi"("report in"=w299, "alignment (default)"=HTML_Report_Image_Alignment."LEFT", "image depth"=w292, "ctrl reference"=w300, "error in (no error)"=w298, "MS Office parameters"=T5 {"position (Excel)"={"row"=14, "column"=0}, "name (Excel)"="", "bookmark (Word)"=""}) -> ("report out"=w290:refnum<class "NI_report.lvclass">, "error out"=w289:errorcluster)  [unwired: 6 in, 2 out]
        n125 = Build Array(w271, w272, w273, w274, w269, w268) -> (w275:string[])
        n126 = for {
          tunnel: w275 -> [w326] mode=indexing
          tunnel: T4 [{"position (Excel)"={"row"=2, "column"=1}, "name (Excel)"="", "bookmark (Word)"=""}, {"position (Excel)"={"row"=3, "column"=1}, "name (Excel)"="", "bookmark (Word)"=""}, {"position (Excel)"={"row"=2, "column"=5}, "name (Excel)"="", "bookmark (Word)"=""}, {"position (Excel)"={"row"=12, "column"=1}, "name (Excel)"="", "bookmark (Word)"=""}, {"position (Excel)"={"row"=3, "column"=5}, "name (Excel)"="", "bookmark (Word)"=""}, {"position (Excel)"={"row"=13, "column"=1}, "name (Excel)"="", "bookmark (Word)"=""}] ("MS Office parameters") -> [w323] mode=indexing
          tunnel: w290 -> [w327]
          tunnel: [w325] -> w288
          tunnel: w289 -> [w328]
          tunnel: [w324] -> w277
          n127 = call-poly <vilib>:"Append Report Text.vi"("report in"=w327, "MS Office parameters"=w323, "text"=w326, "error in (no error)"=w328) -> ("report out"=w325:refnum<class "NI_report.lvclass">, "error out"=w324:errorcluster)  [unwired: 8 in, 2 out]
        }
        n128 = call "File Dialog"("error in"=w277) -> ("selected path"=w283:path, "error out"=w278:errorcluster)  [unwired: 11 in, 2 out]
        n129 = call <vilib>:"Clear Errors.vi"("error in (no error)"=w278) -> ()  [unwired: 5 in, 2 out]
        n130 = Path To String(path=w283) -> (string=w282:string)
        n131 = Concatenate Strings(w282, ".pdf" ("string")) -> (w280:string)
        n132 = String To Path(string=w280) -> (path=w279:path)
        n133 = case shown="False" FALSE {
          tunnel: [w310 w322] -> w302
          tunnel: [w313 w321] -> w301
          tunnel: w288 -> [w311 w320]
          tunnel: w279 -> [w309 w319]
          tunnel: w277 -> [w312 w318]
          frame False {
            w315 = 0 items=["xlTypePDF", "xlTypeXPS"] ("Type")
            n134 = call <vilib>:"Excel Get ActiveX References.vi"("report in"=w311, "error in (no error)"=w312) -> ("report out"=w310:refnum<class "NI_report.lvclass">, "Excel._Worksheet"=w316:refnum<k7>, "error out"=w317:errorcluster)  [unwired: 7 in, 4 out]
            n135 = invoke class="_Worksheet" method="ExportAsFixedFormat"(reference=w316, error in=w317, "Type"=w315, "Filename"=w309, "OpenAfterPublish"=TRUE) -> (error out=w313:errorcluster)  [unwired: 7 in, 11 out]
          }
          frame True {
            n136 = call-dynamic "Save Report to File.vi"("report in"=w320, "report file path"=w319, "error in (no error)"=w318) -> ("report out"=w322:refnum<class "NI_report.lvclass">, "error out"=w321:errorcluster)  [unwired: 11 in]
          }
        }
        n137 = call-dynamic "Dispose Report.vi"("report in"=w302, "error in (no error)"=w301) -> ("error out"=w284:errorcluster)  [unwired: 13 in]
        n138 = flat-sequence {
          tunnel: w284 -> [w329]
          tunnel: [w329] -> w285
          frame #0 {
            n139 = local write "Status bar"("Completed" ("Status bar")) -> ()
          }
        }
      }
    }
    n140 = call <vilib>:"Simple Error Handler.vi"("error in (no error)"=w60) -> ("error out"=w59:errorcluster)  [unwired: 4 in, 4 out]
    n141 = Wait (ms)(milliseconds to wait=u32 500) -> ()  [unwired: 1 out]
  }
  n142 = call <vilib>:"DB Tools Close Connection.vi"("error in (no error)"=w42, "connection reference"=w41) -> ("error out"=w17:errorcluster)  [unwired: 5 in]
  n143 = flat-sequence {
    tunnel: [w338] -> w16
    tunnel: w17 -> [w339]
    frame #0 {
      n144 = property class="App"(error in=w339) -> (error out=w340:errorcluster, "App.Kind"=w341:T17)  [unwired: 1 in, 1 out]
      n145 = case shown="\"Run Time System\"" w341 {
        tunnel: w340 -> [w342 w344]
        tunnel: [w342 w343] -> w338
        frame Default {
        }
        frame "Run Time System" {
          n146 = invoke class="VI" method="FP.Close"(error in=w344) -> (error out=w343:errorcluster)  [unwired: 2 in, 2 out]
        }
      }
    }
  }
  "error out" <- w16
